vi "Resolve Path.vi"(8 "error in (no error)":errorcluster, 11 "Path":path) -> (0 "error out":errorcluster, 3 "Resolved":path)   [LabVIEW 2020, in "vim-liner.lvlib"]
uses:
  vim-liner.lvlib
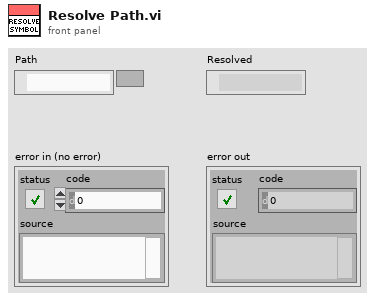
[diagram p1: front panel]
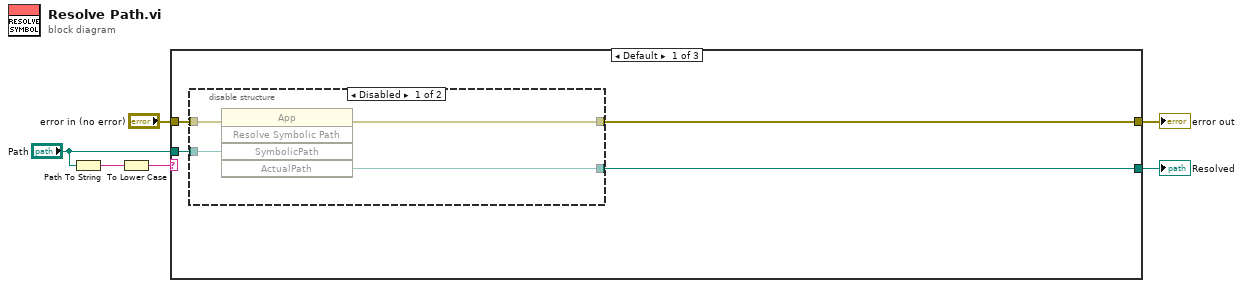
[diagram p0: block diagram]
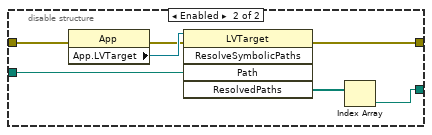
[diagram p2: hidden frame]
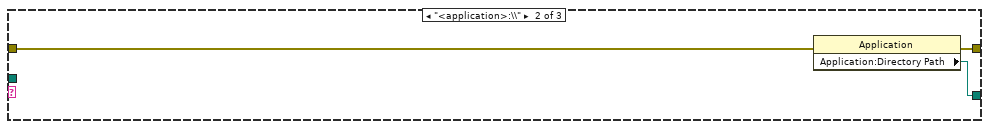
[diagram p3: hidden frame]
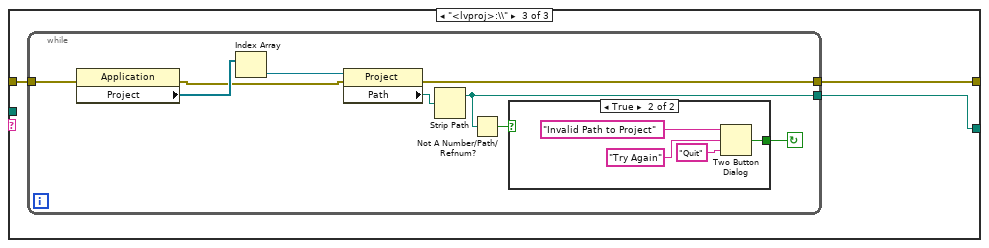
[diagram p4: hidden frame]
diagram:
  n1 = Path To String(path="Path") -> (string=w6:string)
  n2 = To Lower Case(string=w6) -> (all lower case string=w5:string)
  n3 = case shown="Default" w5 {
    tunnel: "Path" -> [w7 _ _]
    tunnel: [w10 w24 w25] -> w2
    tunnel: [w9 w23 w27] -> w3
    tunnel: "error in (no error)" -> [w8 w22 w26]
    frame Default {
      n4 = disable-structure shown="Disabled" {
        disable-tunnel: [w14 w15] -> w10
        disable-tunnel: [w13 w16] -> w9
        disable-tunnel: w8 -> [w12 w20]
        disable-tunnel: w7 -> [w11 w18]
        frame Disabled {
          n5 = invoke class="App" method="Resolve Symbolic Path"(error in=w12, "SymbolicPath"=w11) -> (error out=w13:errorcluster, "ActualPath"=w14:path)  [unwired: 3 in, 3 out]
        }
        frame Enabled {
          n6 = property class="App"(error in=w20) -> (error out=w19:errorcluster, "App.LVTarget"=w21:refnum<vi>)  [unwired: 1 in, 1 out]
          n7 = invoke class="LVTarget" method="ResolveSymbolicPaths"(reference=w21, error in=w19, "Path"=w18) -> (error out=w16:errorcluster, "ResolvedPaths"=w17:path[])  [unwired: 2 in, 3 out]
          n8 = Index Array(array=w17) -> (element=w15:path)  [unwired: 1 in]
        }
      }
    }
    frame "<application>:\\" {
      n9 = property class="Application"(error in=w22) -> (error out=w23:errorcluster, "Application:Directory Path"=w24:path)  [unwired: 1 in, 1 out]
    }
    frame "<lvproj>:\\" {
      n10 = while {
        tunnel: [w33] -> w27
        tunnel: w26 -> [w32]
        tunnel: [w29] -> w25
        stop <- w28 continue-if-true
        n11 = property class="Application"(error in=w32) -> (error out=w34:errorcluster, "Project"=w36:refnum<vi>[])  [unwired: 1 in, 1 out]
        n12 = Index Array(array=w36) -> (element=w35:refnum<vi>)  [unwired: 1 in]
        n13 = property class="Project"(reference=w35, error in=w34) -> (error out=w33:errorcluster, "Path"=w31:path)  [unwired: 1 out]
        n14 = Strip Path(path=w31) -> (stripped path=w29:path)  [unwired: 1 out]
        n15 = Not A Number/Path/Refnum?(number/path/refnum=w29) -> (NaN/Path/Refnum?=w30:bool)
        n16 = case shown="True" w30 {
          tunnel: [_ w37] -> w28
          frame False {
          }
          frame True {
            n17 = Two Button Dialog(message="Invalid Path to Project", 1:"Quit" ("F button name (\"Cancel\")"), 2:"Try Again" ("T button name (\"OK\")")) -> (T button?=w37:bool)
          }
        }
      }
    }
  }
  "error out" <- w3
  "Resolved" <- w2
